vi "Get All Failed Tests.vi"(10 "Raw Results":T1[][](array[typedef]), 11 "Parsed Results Data (by VI)":T4) -> (3 "Failed Tests":T1[](array[typedef]))   [LabVIEW 2019]
uses:
  <vilib>/addons/analyzer/_vianresshared.llb/VIAnRes Parsed Results Data (by VI).ctl
  <vilib>/addons/analyzer/_analyzerctrls.llb/VIAnCtl Results.ctl
  <vilib>/addons/analyzer/_analyzerctrls.llb/VIAnCtl ResultsData (index).ctl
  <vilib>/addons/analyzer/_analyzerctrls.llb/VIAnCtl ResultStatus.ctl
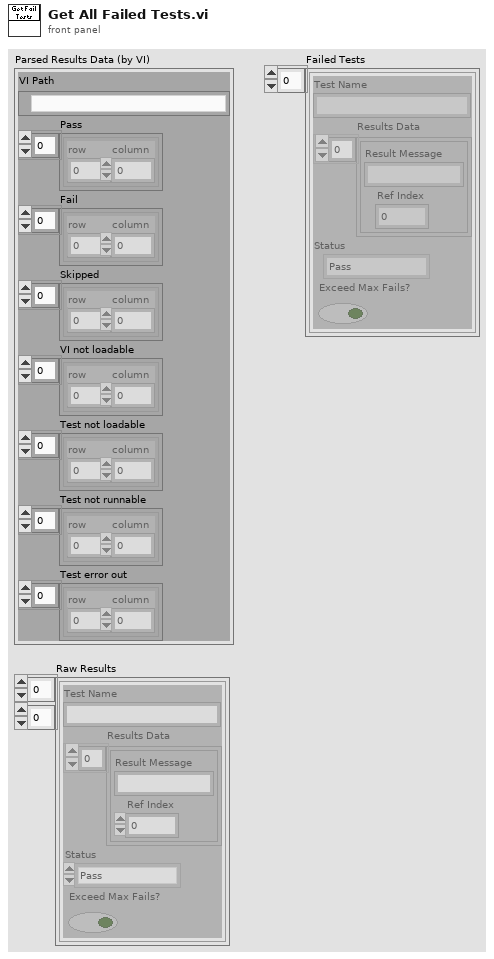
[diagram p1: front panel]
types:
  T1 = typedef "VIAnCtl Results.ctl" = cluster{"Test Name":string, "Results Data":T2[], "Status":T3, "Exceed Max Fails?":bool}
  T2 = typedef "VIAnCtl ResultsData (index).ctl" = cluster{"Result Message":string, "Ref Index":i32}
  T3 = typedef "VIAnCtl ResultStatus.ctl" = enum16{"Pass", "Fail", "Skipped", "VI not loadable", "Test not loadable", "Test not runnable", "Test error out"}
  T4 = typedef "VIAnRes Parsed Results Data (by VI).ctl" = cluster{"VI Path":path, "Pass":cluster{"row":i32, "column":i32}[], "Fail":cluster{"row":i32, "column":i32}[], "Skipped":cluster{"row":i32, "column":i32}[], "VI not loadable":cluster{"row":i32, "column":i32}[], "Test not loadable":cluster{"row":i32, "column":i32}[], "Test not runnable":cluster{"row":i32, "column":i32}[], "Test error out":cluster{"row":i32, "column":i32}[]}
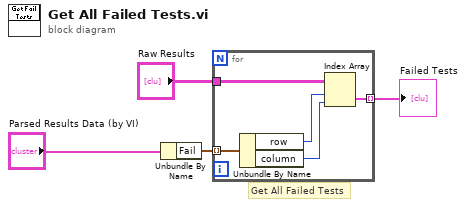
[diagram p0: block diagram]
diagram:
  # "Get All Failed Tests"
  n1 = Unbundle By Name("Parsed Results Data (by VI)") -> ("Fail"=w1:cluster{"row":i32, "column":i32}[])
  n2 = for {
    tunnel: w1 -> [w8] mode=indexing
    tunnel: "Raw Results" -> [w9]
    tunnel: [w5] -> w3 mode=indexing
    n3 = Unbundle By Name(w8) -> ("row"=w7:i32, "column"=w6:i32)
    n4 = Index Array(array=w9, index (row)=w7, index (col)=w6) -> (element=w5:T1)
  }
  "Failed Tests" <- w3
